vi "Manage Current Function.vi"(7 "Action":enum16{"Get", "Set"}(ring), 8 "error in (no error)":errorcluster, 11 "Set Function":T1) -> (0 "error out":errorcluster, 3 "Get Function":T1)   [LabVIEW 2020]
doc: "This FGV stores the last-selected function from the menu controls. It is a simple memory for the application."
uses:
  Controls/Function.ctl
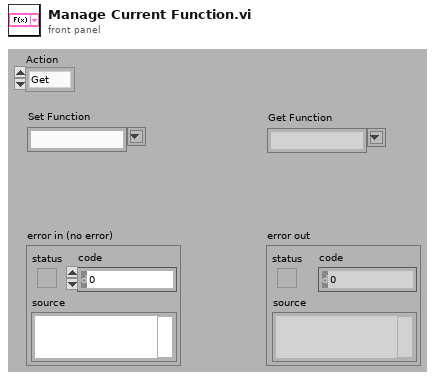
[diagram p1: front panel]
types:
  T1 = typedef "Function.ctl" = string
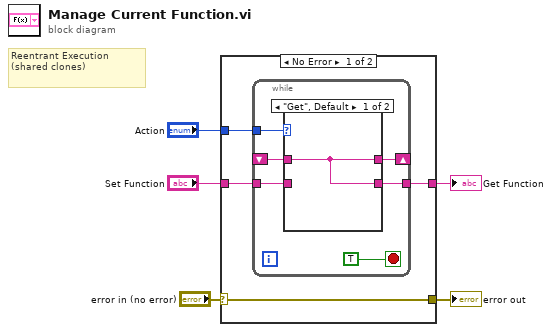
[diagram p0: block diagram]
diagram:
  # "Reentrant Execution\n(shared clones)"
  n1 = case shown="No Error" "error in (no error)" {
    selector: "error in (no error)" -> [w6 w19]
    tunnel: "Action" -> [w9 _]
    tunnel: "Set Function" -> [w8 w18]
    tunnel: [w7 w18] -> w3
    tunnel: [w6 w19] -> w1
    frame No Error {
      n2 = while {
        tunnel: w9 -> [w15]
        shift-right: [w13] -> _
        shift-left: _ -> [w14]
        tunnel: w8 -> [w12]
        tunnel: [w11] -> w7
        stop <- TRUE stop-if-true
        n3 = case shown="\"Get\", Default" w15 {
          tunnel: w14 -> [w16 _]
          tunnel: [w16 w17] -> w13
          tunnel: w12 -> [_ w17]
          tunnel: [w16 w17] -> w11
          frame "Get", Default {
          }
          frame "Set" {
          }
        }
      }
    }
    frame Error {
    }
  }
  "Get Function" <- w3
  "error out" <- w1
